vi "Collector.vi"(6 "MotorSpeed":dbl, 7 "Action":T10, 8 "Error in":errorcluster, 9 "BottomLS":T8={"DevStatus"={"status"=FALSE, "code"=0, "source"=""}, "DIO Channel"=enum."Invalid", "Digital Module"=enum."Digital Module 1"}, 10 "TopLS":T8={"DevStatus"={"status"=FALSE, "code"=0, "source"=""}, "DIO Channel"=enum."Invalid", "Digital Module"=enum."Digital Module 1"}, 11 "Motor":T1={"DeviceStatus"={"status"=FALSE, "code"=0, "source"=""}, "Type"=enum."PWM", "PWM"={"Digital Module"=enum."Digital Module 1", "PWM Channel"=enum."Invalid", "DeadBand"={"Name"="", "maxPositivePwm"=0, "minPositivePwm"=0, "centerPwm"=0, "maxNegativePwm"=0, "minNegativePwm"=0, "angularRange"=0}}, "CAN"={"Device Number"=0, "Control Mode"=enum."Percent VBus", "Semaphore"=refnum, "Max Vout"=12.0}, "Invert"=FALSE, "TransformRef"=refnum, "InvTransformRef"=refnum}) -> (0 "Error out":errorcluster, 1 "Lower Triggered?":bool, 2 "Upper Triggered?":bool)   [LabVIEW 2013]
doc: "Controls the collector arm, along with the two sets of limit switches associated with it (one set all the way up, the other all the way down). NOTE: all states return the status of the limit switches. It has the following actions:\n-Init: takes references to the motor and limit switches and stores them in shift registers\n-Raise: attempts to raise the collector (nothing happens if the upper limit switch is triggered)\n-Lower: attempts to lower the collector (nothing happens if the lower limit switch is triggered)\n-Stop: stops the motor\n-GetStatus: returns the value of the limit switches"
uses:
  CollectorAction.ctl
  <vilib>/Rock Robotics/WPI/DigitalInput/WPI_DigitalInputDevRef.ctl
  <vilib>/Rock Robotics/SystemInterfaces/DIO/FPGA_DIOChannel.ctl
  <vilib>/Rock Robotics/SystemInterfaces/Typedef/FPGA_TypedefDigitalModule.ctl
  <vilib>/Rock Robotics/WPI/MotorControl/WPI_MotorControlDeviceRef.ctl
  <vilib>/Rock Robotics/SystemInterfaces/DIO/FPGA_DIOPWMChannel.ctl
  <vilib>/Rock Robotics/WPI/PWM/WPI_PWMDeadband.ctl
  <vilib>/Rock Robotics/WPI/CAN/Jaguar/SubVIs/WPI_CANJaguar_ControlMode.ctl
  <vilib>/Rock Robotics/WPI/PWM/WPI_PWMTransform_ConPane.ctl
panel:
  in  "MotorSpeed 2":dbl
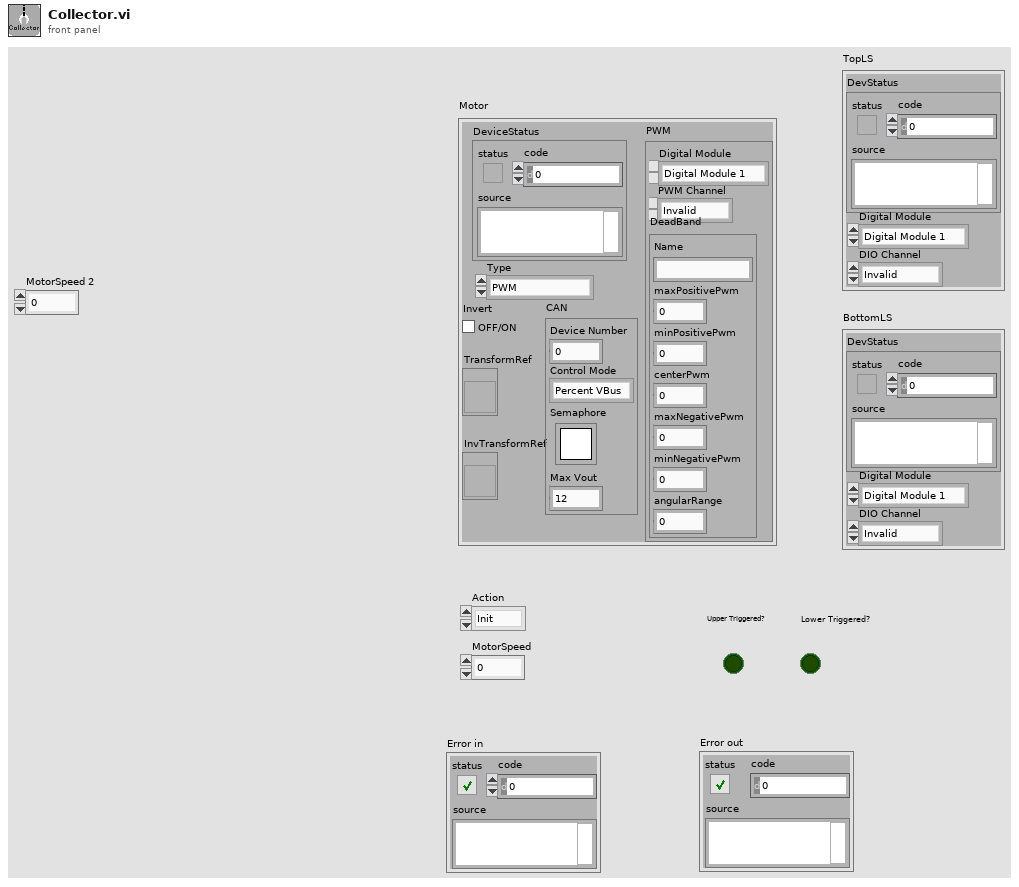
[diagram p1: front panel]
types:
  T1 = typedef "WPI_MotorControlDeviceRef.ctl" = cluster{"DeviceStatus":errorcluster, "Type":enum16{"PWM", "CAN"}, "PWM":cluster{"Digital Module":T2, "PWM Channel":T3, "DeadBand":T4}, "CAN":cluster{"Device Number":u8, "Control Mode":T5, "Semaphore":T6, "Max Vout":dbl}, "Invert":bool, "TransformRef":T7, "InvTransformRef":T7}
  T2 = typedef "FPGA_TypedefDigitalModule.ctl" = enum16{"Digital Module 1", "Digital Module 2"}
  T3 = typedef "FPGA_DIOPWMChannel.ctl" = enum8{"PWM 1", "PWM 2", "PWM 3", "PWM 4", "PWM 5", "PWM 6", "PWM 7", "PWM 8", "PWM 9", "PWM 10", "Invalid"}
  T4 = typedef "WPI_PWMDeadband.ctl" = cluster{"Name":string, "maxPositivePwm":i32, "minPositivePwm":i32, "centerPwm":i32, "maxNegativePwm":i32, "minNegativePwm":i32, "angularRange":u16}
  T5 = typedef "WPI_CANJaguar_ControlMode.ctl" = enum8{"Percent VBus", "Current", "Speed", "Position", "Voltage"}
  T6 = typedef "Semaphore RefNum" = refnum<k1>
  T7 = typedef "WPI_PWMTransform_ConPane.ctl" = refnum<vi>
  T8 = typedef "WPI_DigitalInputDevRef.ctl" = cluster{"DevStatus":errorcluster, "DIO Channel":T9, "Digital Module":T2}
  T9 = typedef "FPGA_DIOChannel.ctl" = enum8{"DIO 1", "DIO 2", "DIO 3", "DIO 4", "DIO 5", "DIO 6", "DIO 7", "DIO 8", "DIO 9", "DIO 10", "DIO 11", "DIO 12", "DIO 13", "DIO 14", "Invalid"}
  T10 = typedef "CollectorAction.ctl" = enum16{"Init", "Raise", "Lower", "Stop", "GetStatus"}
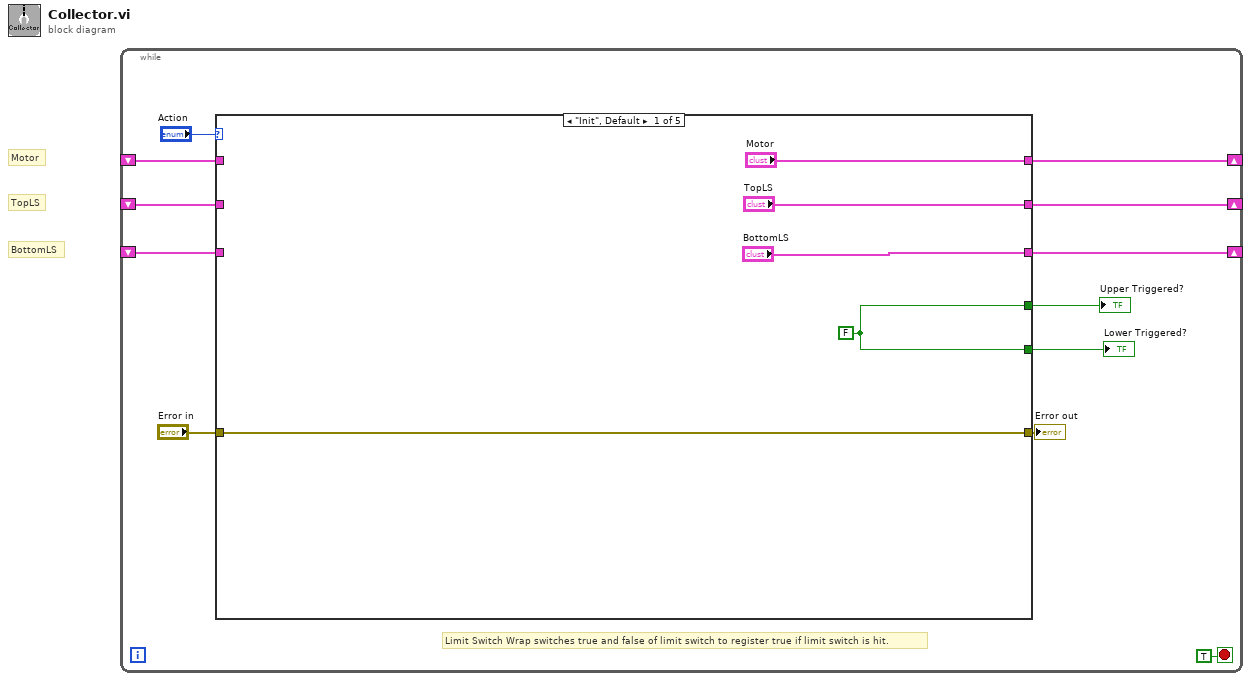
[diagram p0: block diagram]
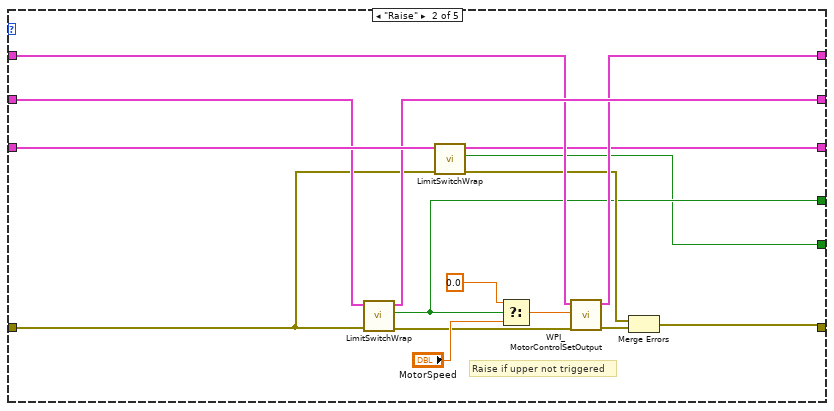
[diagram p2: hidden frame]
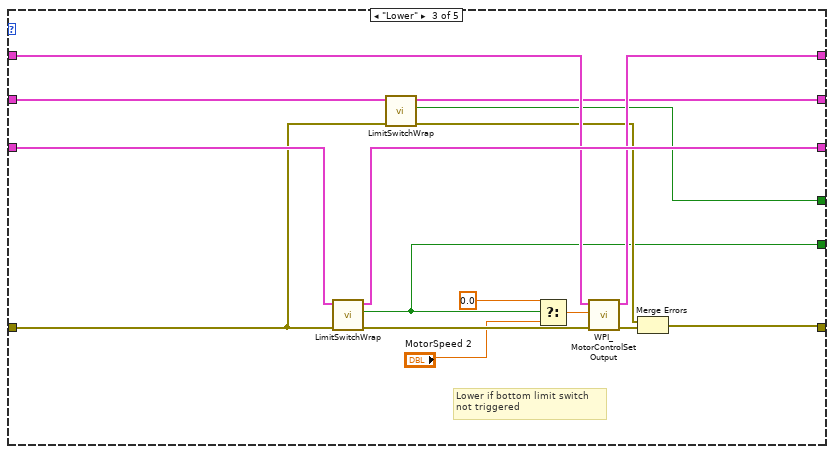
[diagram p3: hidden frame]
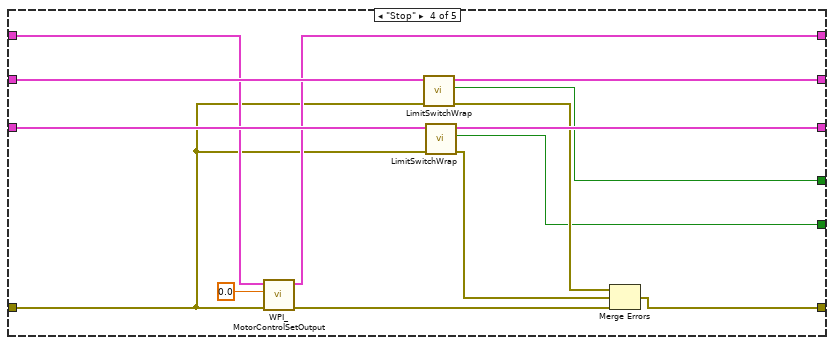
[diagram p4: hidden frame]
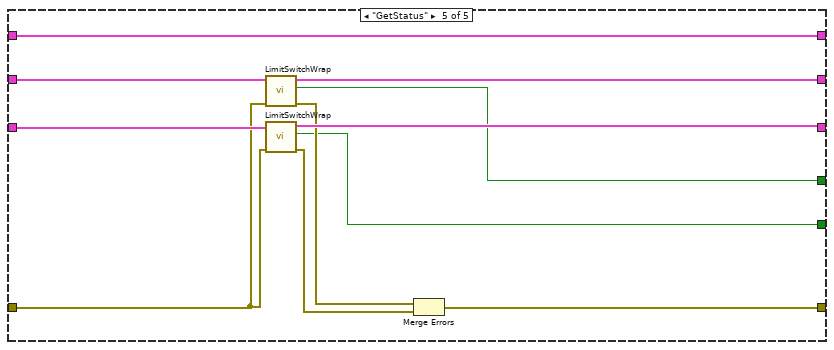
[diagram p5: hidden frame]
diagram:
  # "BottomLS"
  # "TopLS"
  # "Motor"
  n1 = while {
    shift-right: [w9] -> _
    shift-left: _ -> [w6]
    shift-right: [w10] -> _
    shift-left: _ -> [w7]
    shift-right: [w11] -> _
    shift-left: _ -> [w8]
    stop <- TRUE stop-if-true
    # "Limit Switch Wrap switches true and false of limit switch to register true if limit switch is hit."
    n2 = case shown="\"Init\", Default" "Action" {
      tunnel: ["Motor" w25 w42 w59 w74] -> w11
      tunnel: ["TopLS" w27 w41 w57 w71] -> w10
      tunnel: ["BottomLS" w24 w45 w58 w70] -> w9
      tunnel: w8 -> [_ w26 w43 w60 w74]
      tunnel: w7 -> [_ w28 w49 w62 w72]
      tunnel: w6 -> [_ w33 w46 w61 w73]
      tunnel: "Error in" -> [w17 w23 w40 w56 w69]
      tunnel: [w17 w21 w39 w54 w66] -> w4
      tunnel: [w13 w18 w35 w51 w65] -> w1
      tunnel: [w13 w19 w36 w50 w64] -> w2
      frame "Init", Default {
        w13 = FALSE
      }
      frame "Raise" {
        # "Raise if upper not triggered"
        n3 = call "LimitSwitchWrap.vi"("error in"=w23, "DigitalInputDevRef"=w28) -> ("error out"=w29:errorcluster, "Triggered"=w19:bool, "DigitalInputDevRef 2"=w27:T8)  [unwired: 7 in]
        n4 = call "LimitSwitchWrap.vi"("error in"=w23, "DigitalInputDevRef"=w33) -> ("error out"=w20:errorcluster, "Triggered"=w18:bool, "DigitalInputDevRef 2"=w24:T8)  [unwired: 7 in]
        n5 = Select(t=0.0, s=w19, f="MotorSpeed") -> (s? t:f=w32:dbl)
        n6 = call <vilib>:"WPI_MotorControlSetOutput.vi"("error in (no error)"=w29, "Output"=w32, "MotorControlDevRef"=w26) -> ("error out"=w22:errorcluster, "MotorControlDevRef"=w25:T1)  [unwired: 6 in, 1 out]
        n7 = Merge Errors(w20, w22) -> (w21:errorcluster)
      }
      frame "Lower" {
        # "Lower if bottom limit switch\nnot triggered"
        n8 = call "LimitSwitchWrap.vi"("error in"=w40, "DigitalInputDevRef"=w46) -> ("error out"=w44:errorcluster, "Triggered"=w35:bool, "DigitalInputDevRef 2"=w45:T8)  [unwired: 7 in]
        n9 = call "LimitSwitchWrap.vi"("error in"=w40, "DigitalInputDevRef"=w49) -> ("error out"=w37:errorcluster, "Triggered"=w36:bool, "DigitalInputDevRef 2"=w41:T8)  [unwired: 7 in]
        n10 = Select(t=0.0, s=w35, f="MotorSpeed 2") -> (s? t:f=w48:dbl)
        n11 = call <vilib>:"WPI_MotorControlSetOutput.vi"("error in (no error)"=w44, "Output"=w48, "MotorControlDevRef"=w43) -> ("error out"=w38:errorcluster, "MotorControlDevRef"=w42:T1)  [unwired: 6 in, 1 out]
        n12 = Merge Errors(w37, w38) -> (w39:errorcluster)
      }
      frame "Stop" {
        n13 = call <vilib>:"WPI_MotorControlSetOutput.vi"("error in (no error)"=w56, "Output"=0.0, "MotorControlDevRef"=w60) -> ("error out"=w55:errorcluster, "MotorControlDevRef"=w59:T1)  [unwired: 6 in, 1 out]
        n14 = call "LimitSwitchWrap.vi"("error in"=w56, "DigitalInputDevRef"=w62) -> ("error out"=w52:errorcluster, "Triggered"=w50:bool, "DigitalInputDevRef 2"=w57:T8)  [unwired: 7 in]
        n15 = call "LimitSwitchWrap.vi"("error in"=w56, "DigitalInputDevRef"=w61) -> ("error out"=w53:errorcluster, "Triggered"=w51:bool, "DigitalInputDevRef 2"=w58:T8)  [unwired: 7 in]
        n16 = Merge Errors(w52, w53, w55) -> (w54:errorcluster)
      }
      frame "GetStatus" {
        n17 = call "LimitSwitchWrap.vi"("error in"=w69, "DigitalInputDevRef"=w72) -> ("error out"=w67:errorcluster, "Triggered"=w64:bool, "DigitalInputDevRef 2"=w71:T8)  [unwired: 7 in]
        n18 = call "LimitSwitchWrap.vi"("error in"=w69, "DigitalInputDevRef"=w73) -> ("error out"=w68:errorcluster, "Triggered"=w65:bool, "DigitalInputDevRef 2"=w70:T8)  [unwired: 7 in]
        n19 = Merge Errors(w67, w68) -> (w66:errorcluster)
      }
    }
    "Error out" <- w4
    "Upper Triggered?" <- w2
    "Lower Triggered?" <- w1
  }
